vi "SeriellRead_ECD.vi"(5 "Port4":string, 6 "SkalierungsfaktorHorst":dbl[](array[numeric]), 7 "VorwortHorst":string[](array[string]), 8 "error in":errorcluster, 9 "Zwischenspeicher":string[](array[string]), 10 "Senden?":bool[](array[boolean]), 11 "FPGA-VI-Referenz (Ausgang)":refnum<k20>) -> (0 "Port4":string, 1 "Senden?":bool[](array[boolean]), 2 "Zwischenspeicher":string[](array[string]), 3 "error out":errorcluster)   [LabVIEW 2017]
uses:
  <vilib>/Utility/error.llb/Error Cluster From Error Code.vi
  <vilib>/rvi/errors/niLvFpgaAdjustHostInterfaceError.vi
  GVECDs_ECD.vi
  <vilib>/rvi/interface/nirviMethod/nirviMethod.xnode
  FPGA Bitfiles/HAGAR-V_FPGATargetECD_FPGA-ProgrammECD_LbBtUh8SPQY.lvbitx
  FPGA_ECD/FPGA-Programm_ECD.vi
  <vilib>/rvi/errors/niLvFpgaMergeErrorWithErrorCode.vi
  <vilib>/FPGAPlugInAG/cRIO-9035/niLvFpga_ReadFifo_cRIO-9035.vi
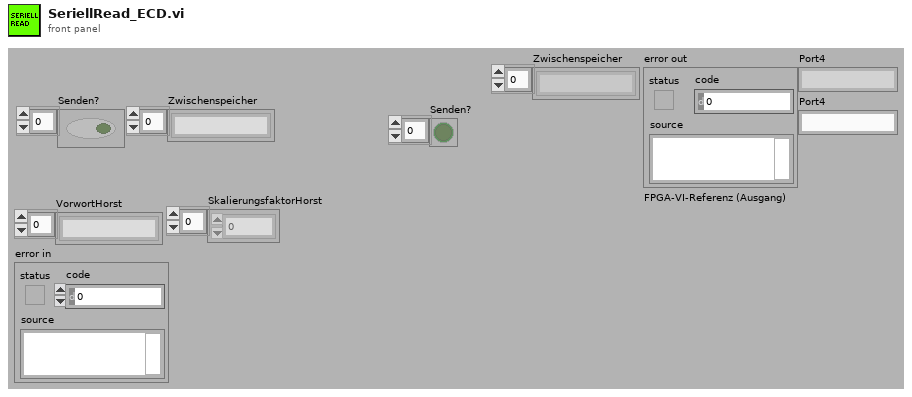
[diagram p1: front panel]
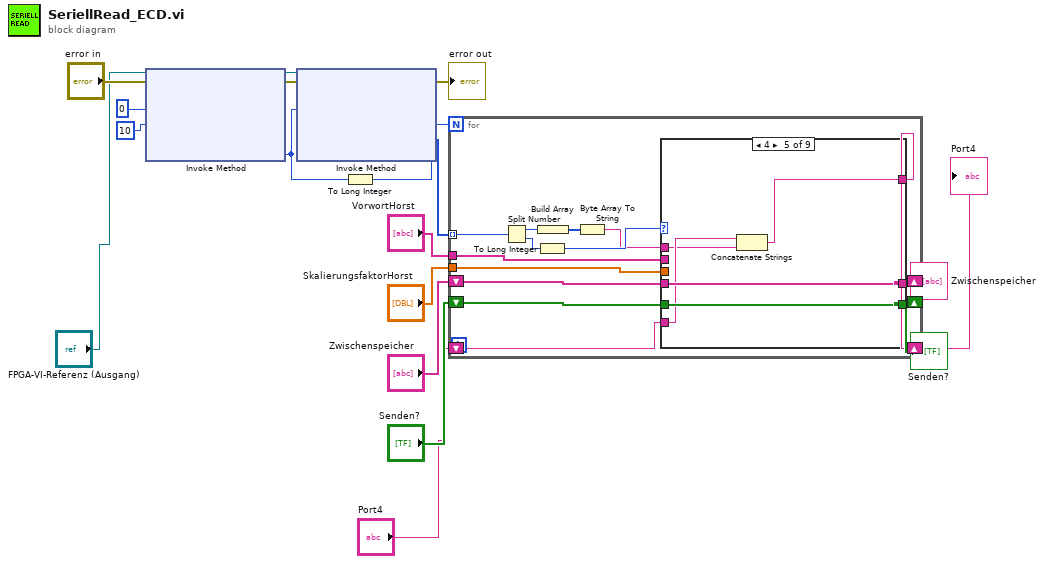
[diagram p0: block diagram]
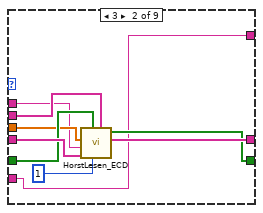
[diagram p3: hidden frame]
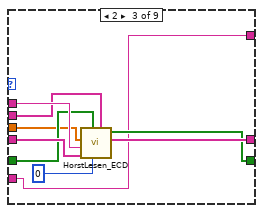
[diagram p4: hidden frame]
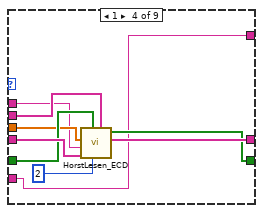
[diagram p5: hidden frame]
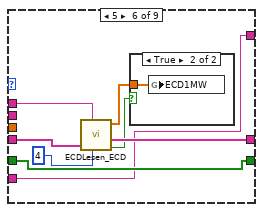
[diagram p6: hidden frame]
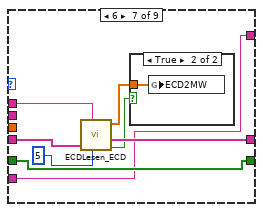
[diagram p8: hidden frame]
diagram:
  n1 = xnode "Invoke Method"("FPGA-VI-Referenz (Eingang)"="FPGA-VI-Referenz (Ausgang)", "Fehler (Eingang)"="error in", "Anzahl der Elemente"=u32 0 ("Number of Elements"), "Timeout (ms)"=10) -> ("FPGA-VI-Referenz (Ausgang)"=w14:refnum<k20>, "Fehler (Ausgang)"=w5:errorcluster, "Verbleibende Elemente"=w17:u32)  [unwired: 1 out]
  n2 = xnode "Invoke Method"("FPGA-VI-Referenz (Eingang)"=w14, "Fehler (Eingang)"=w5, "Anzahl der Elemente"=w17) -> ("Fehler (Ausgang)"=→"error out":errorcluster, "Daten"=w13:u16[])  [unwired: 1 in, 2 out]
  n3 = To Long Integer(number=w17) -> (32bit integer=w18:i32)
  n4 = for {
    N: w18 -> [_]
    tunnel: w13 -> [w32] mode=indexing
    shift-right: [w29] -> w10
    shift-left: "Senden?" -> [w28]
    shift-right: [w30] -> w9
    shift-left: "Zwischenspeicher" -> [w31]
    tunnel: "VorwortHorst" -> [w24]
    tunnel: "SkalierungsfaktorHorst" -> [w23]
    shift-right: [w19] -> w2
    shift-left: "Port4" -> [w20]
    n5 = Split Number(x=w32) -> (hi(x)=w27:u8, lo(x)=w25:u8)
    n6 = To Long Integer(number=w25) -> (32bit integer=w22:i32)
    n7 = Build Array(w27) -> (w26:u8[])
    n8 = Byte Array To String(unsigned byte array=w26) -> (string=w21:string)
    n9 = case shown="4" w22 {
      tunnel: w21 -> [_ w37 w53 w55 w64 w75 w84 _ _]
      tunnel: w31 -> [w35 w44 w52 w62 w67 w74 w83 w87 w90]
      tunnel: [w35 w43 w51 w61 w67 w73 w82 w87 w90] -> w30
      tunnel: [w34 w42 w50 w60 w66 w69 w78 w88 w91] -> w29
      tunnel: w28 -> [w34 w41 w49 w59 w66 w69 w78 w88 w91]
      tunnel: w24 -> [_ w40 w48 w58 _ _ _ _ _]
      tunnel: w23 -> [_ w39 w47 w57 _ _ _ _ _]
      tunnel: w20 -> [w33 w36 w45 w54 w65 w68 w77 w86 w89]
      tunnel: [w33 w36 w45 w54 w63 w68 w77 w86 w89] -> w19
      frame 0, Default {
      }
      frame 3 {
        n10 = call "HorstLesen_ECD.vi"("VorwortHorst"=w40, "Port"=1, "Senden?"=w41, "Zwischenspeicher"=w44, "string"=w37, "SkalierungsfaktorHorst"=w39) -> ("Zwischenspeicher"=w43:string[], "Senden?"=w42:bool[])  [unwired: 4 in]
      }
      frame 2 {
        n11 = call "HorstLesen_ECD.vi"("VorwortHorst"=w48, "Port"=0, "Senden?"=w49, "Zwischenspeicher"=w52, "string"=w53, "SkalierungsfaktorHorst"=w47) -> ("Zwischenspeicher"=w51:string[], "Senden?"=w50:bool[])  [unwired: 4 in]
      }
      frame 1 {
        n12 = call "HorstLesen_ECD.vi"("VorwortHorst"=w58, "Port"=2, "Senden?"=w59, "Zwischenspeicher"=w62, "string"=w55, "SkalierungsfaktorHorst"=w57) -> ("Zwischenspeicher"=w61:string[], "Senden?"=w60:bool[])  [unwired: 4 in]
      }
      frame 4 {
        n13 = Concatenate Strings(w65, w64) -> (w63:string)
      }
      frame 5 {
        n14 = call "ECDLesen_ECD.vi"("string"=w75, "Zwischenspeicher"=w74, "Port"=4) -> ("ECDMW"=w71:dbl[], "Zwischenspeicher"=w73:string[], "ECDEmpfangen?"=w72:bool)  [unwired: 3 in]
        n15 = case shown="True" w72 {
          tunnel: w71 -> [_ w76]
          frame False {
          }
          frame True {
            n16 = global write "GVECDs_ECD.vi" "ECD1MW"(w76) -> ()
          }
        }
      }
      frame 6 {
        n17 = call "ECDLesen_ECD.vi"("string"=w84, "Zwischenspeicher"=w83, "Port"=5) -> ("ECDMW"=w80:dbl[], "Zwischenspeicher"=w82:string[], "ECDEmpfangen?"=w81:bool)  [unwired: 3 in]
        n18 = case shown="True" w81 {
          tunnel: w80 -> [_ w85]
          frame False {
          }
          frame True {
            n19 = global write "GVECDs_ECD.vi" "ECD2MW"(w85) -> ()
          }
        }
      }
      frame 7 {
      }
      frame 8 {
      }
    }
  }
  "Senden?" <- w10
  "Zwischenspeicher" <- w9
  "Port4" <- w2
